vi "Check Channel Pair (SubVI).vi"(5 "milliseconds to wait":u32=100, 7 "Test Value":dbl, 8 "error in (no error)":errorcluster, 9 "Input Channel":string, 10 "Output Channel":string, 11 "WorkspaceManager in":T1) -> (0 "error out":errorcluster, 1 "InputChannel Value":dbl, 2 "OutputChannel Value":dbl, 3 "WorkspaceManager out":T1)   [LabVIEW 2019, in "Scalar Channels Testing.lvclass"]
uses:
  Scalar Channels Testing.lvclass
  <vilib>/NI VeriStand/Execution/Workspace/WorkspaceAPI.ctl
  NationalInstruments.VeriStand.ClientAPI
  2b7be6cf-6769-4a88-b00e-7ca73b91b3ba.vi
  <vilib>/NI VeriStand/Execution/Workspace/NI VeriStand - Set Single Channel Value.vi
  <vilib>/NI VeriStand/Execution/Workspace/NI VeriStand - Get Single Channel Value.vi
  <vilib>/NI VeriStand/Execution/Workspace/NI_VS Workspace ExecutionAPI.lvlib
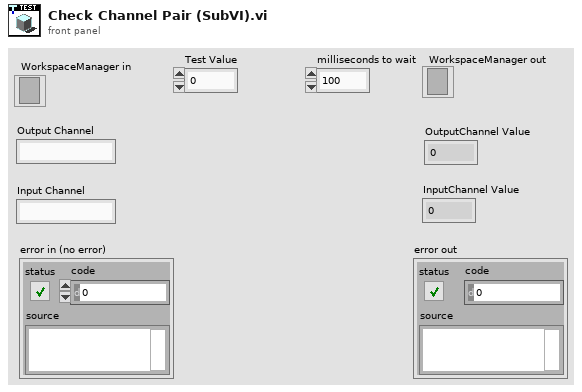
[diagram p1: front panel]
types:
  T1 = typedef "NI_VS Workspace ExecutionAPI.lvlib/WorkspaceAPI.ctl" = refnum<k24>
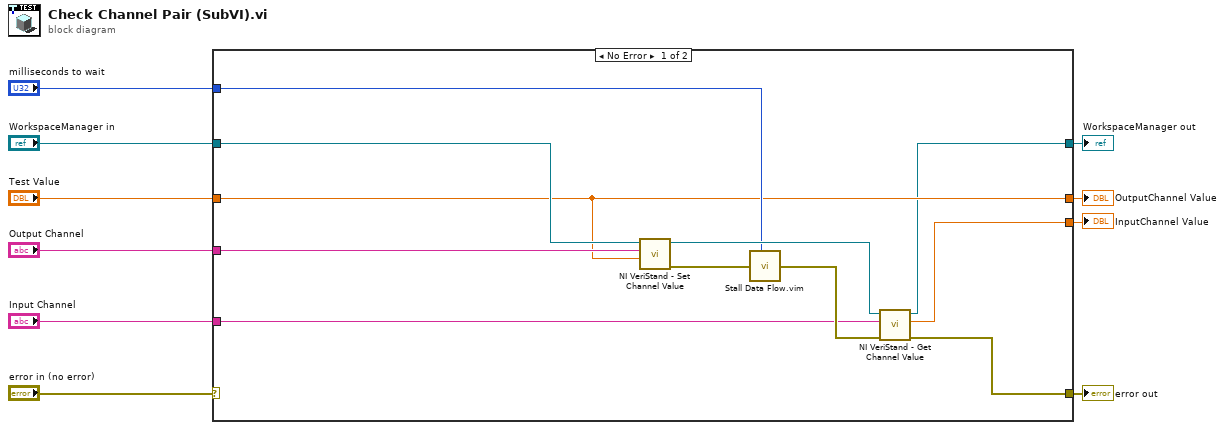
[diagram p0: block diagram]
diagram:
  n1 = case shown="No Error" "error in (no error)" {
    selector: "error in (no error)" -> [_ w24]
    tunnel: [w14 w24] -> w10
    tunnel: "Test Value" -> [w13 w22]
    tunnel: "Input Channel" -> [w18 _]
    tunnel: "Output Channel" -> [w17 _]
    tunnel: "milliseconds to wait" -> [w16 _]
    tunnel: "WorkspaceManager in" -> [w15 w23]
    tunnel: [w13 w22] -> w3
    tunnel: [w12 _] -> w2
    tunnel: [w11 w23] -> w1
    frame No Error {
      n2 = call-poly <vilib>:"NI VeriStand - Set Channel Value.vi"("Value"=w13, "Channel"=w17, "WorkspaceManager in"=w15) -> ("error out"=w20:errorcluster, "WorkspaceManager out"=w19:T1)  [unwired: 7 in]
      n3 = call "Stall Data Flow.vim"("value in"=w20, "milliseconds to wait"=w16) -> ("value out"=w21:errorcluster)  [unwired: 1 out]
      n4 = call-poly <vilib>:"NI VeriStand - Get Channel Value.vi"("error in (no error)"=w21, "Channel"=w18, "WorkspaceManager in"=w19) -> ("error out"=w14:errorcluster, "Value"=w12:dbl, "WorkspaceManager out"=w11:T1)  [unwired: 6 in]
    }
    frame Error {
    }
  }
  "error out" <- w10
  "OutputChannel Value" <- w3
  "InputChannel Value" <- w2
  "WorkspaceManager out" <- w1
